vi "Get generated report  n log in sql.vi"() -> ()   [LabVIEW 2017]
uses:
  SQL/SQL/SQL_DB-Enum.ctl
  Detailed Report/Controls/Detailed_Reports_Columns.ctl
  <vilib>/Utility/error.llb/whitespace.ctl
  <vilib>/Utility/file.llb/Read Delimited Spreadsheet (string).vi
  <vilib>/addons/database/Auxilliary.llb/DB Tools DataTypes.ctl
  <vilib>/addons/database/NI_Database_API.lvlib
  SQL/Detailed Report _Colums_Informatin.ctl
  <vilib>/addons/database/Auxilliary.llb/DB Tools Parameter Dir.ctl
  <vilib>/addons/database/Auxilliary.llb/DB Tools Parameter Info.ctl
panel:
  out "error in (no error) 3":errorcluster
  out "Array":T1(array[cluster])
  in  "time stamp":timestamp
  out "Data out 2":string[][](array[string])
  out "Table/Columns":string[](array[string])
  out "size(s) 3":i32
  out "size(s) 2":i32
  out "size(s)":i32[](array[numeric])
  out "error in (no error) 2":errorcluster
  in  "error in (no error)":errorcluster
  in  "file path (dialog if empty)":path
  out "Serial Number":string
  out "Result for SQl Without Header 2":string[][](array[string])
  out "Result wiht Header 2":string[][](array[string])
  in  "User Name 2":string="mmk"
  in  "Shift 2":string="A"
  in  "Test Type 2":string="Test type"
  in  "Excepted Value 2":string="Excepted Value"
  out "Application Verision":string
  out "Variant":string
  out "Model":string
  out "all rows 2":string[][](array[string])
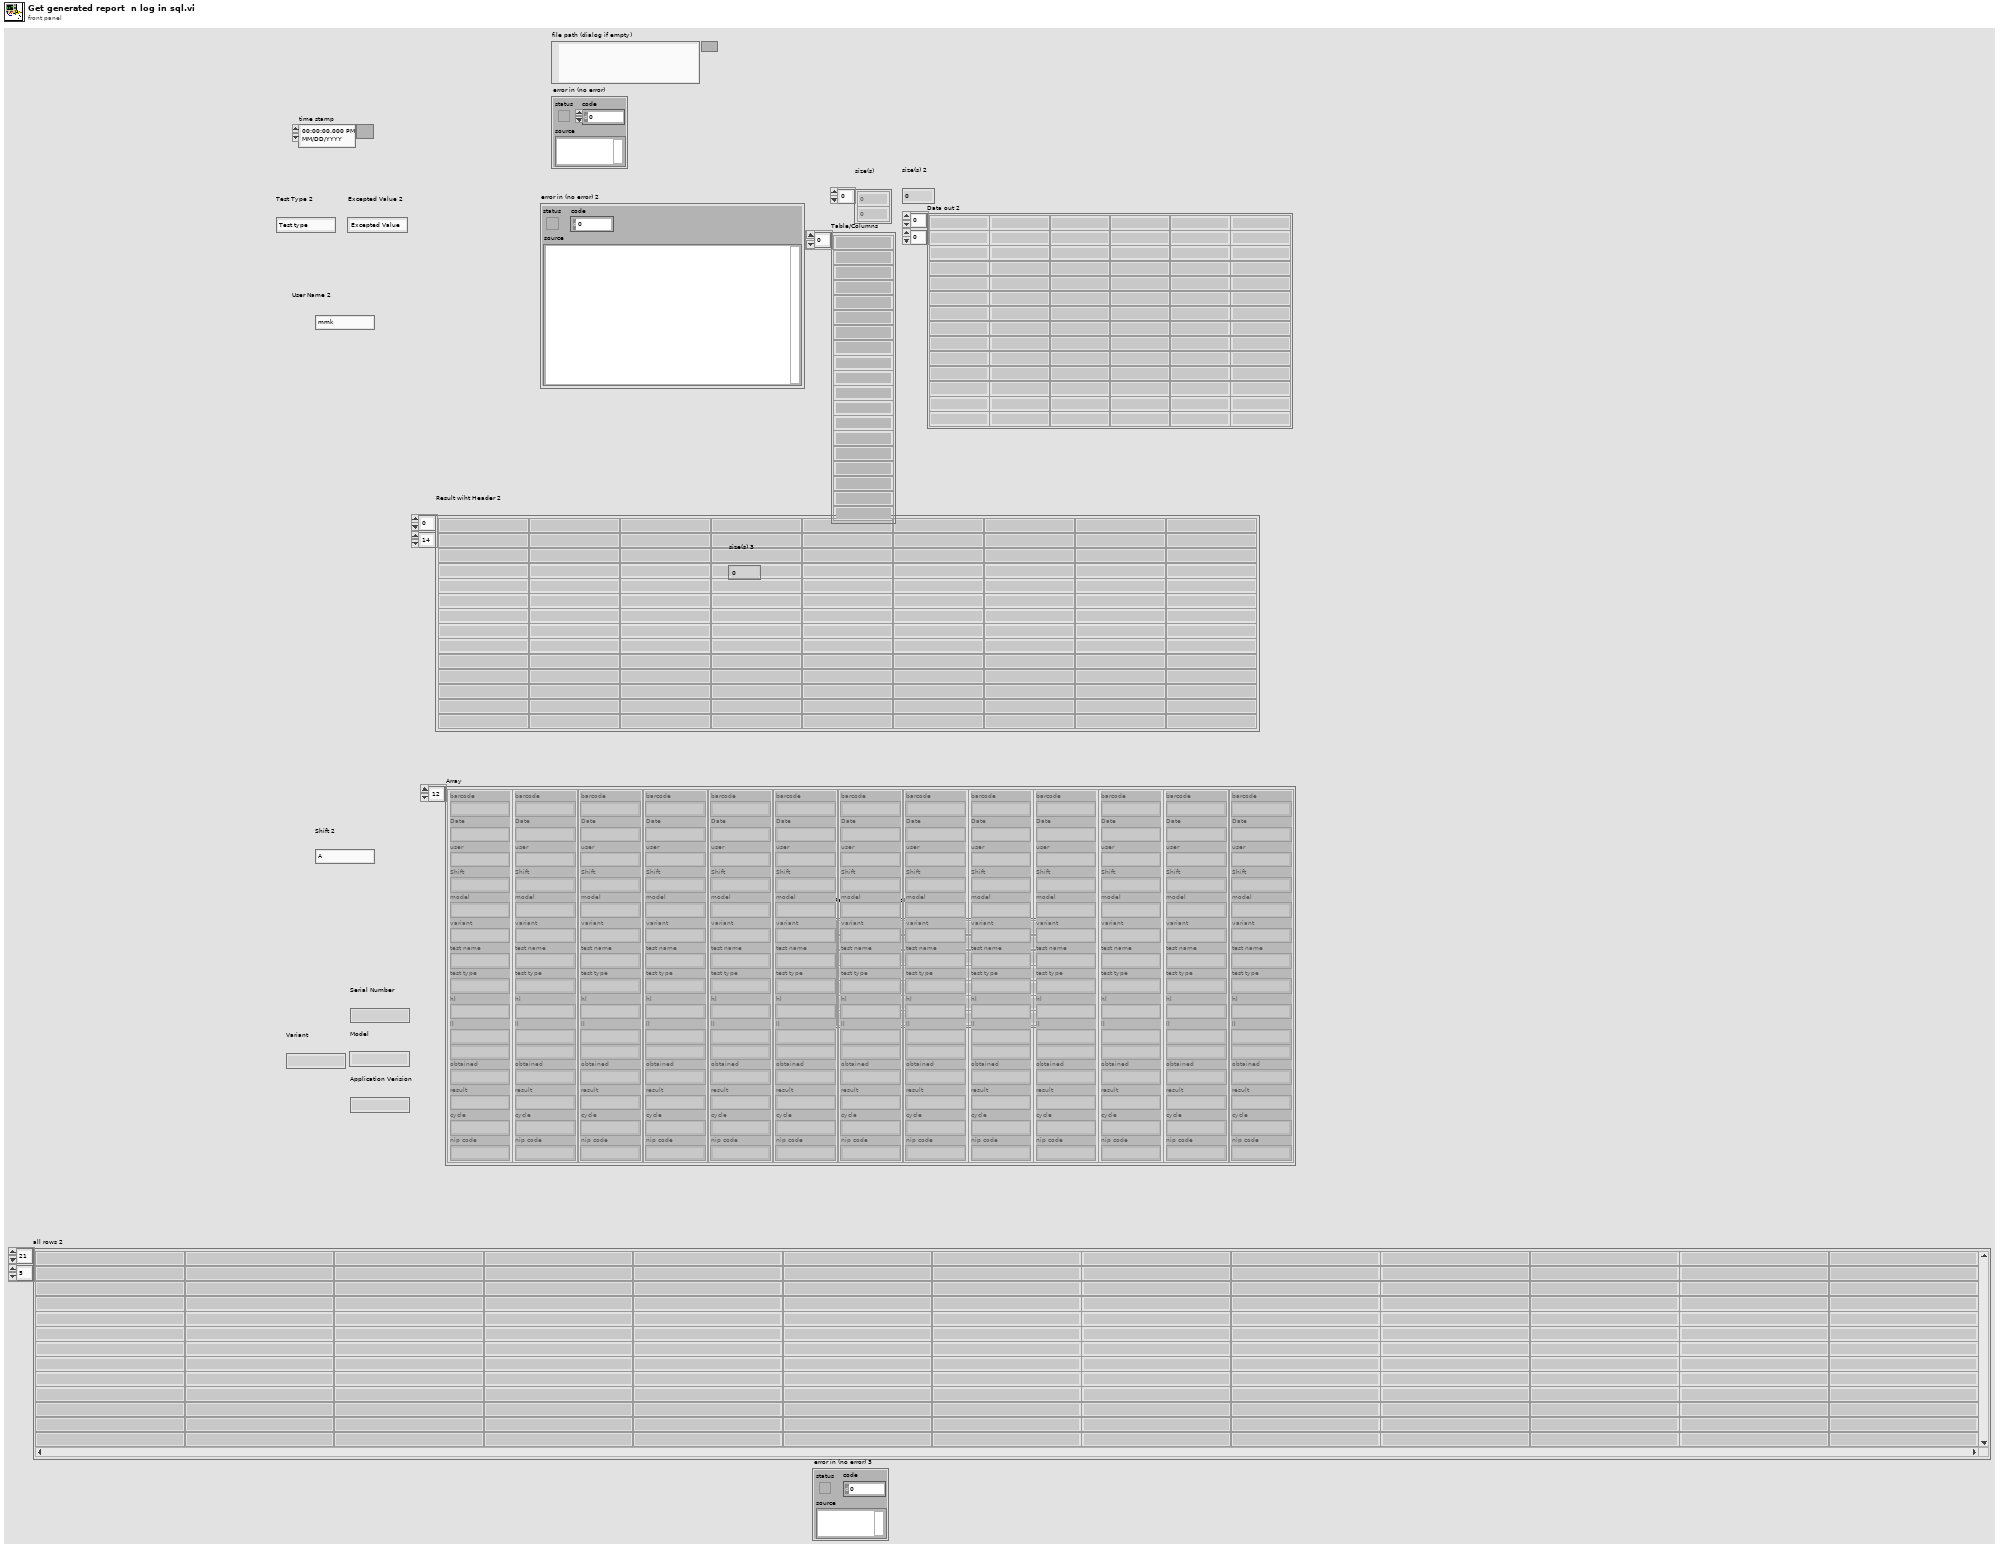
[diagram p1: front panel]
types:
  T1 = cluster{"barcode":string, "Date":string, "user":string, "Shift":string, "model":string, "variant":string, "test name":string, "test type":string, "hl":string, "ll":string, string, "obtained":string, "result":string, "cycle":string, "nip code":string}[]
  T2 = typedef "NI_Database_API.lvlib/DB Tools Parameter Info.ctl" = cluster{"parameter name":string, "type":T3, "direction":T4, "value":variant}
  T3 = typedef "NI_Database_API.lvlib/DB Tools DataTypes.ctl" = enum16{"String", "Long (I32)", "Single (SGL)", "Double (DBL)", "Date/Time", "Binary"}
  T4 = typedef "NI_Database_API.lvlib/DB Tools Parameter Dir.ctl" = enum32{"Input", "Output", "Input/Output", "Return Value"}
  T5 = typedef "SQL_DB-Enum.ctl" = enum16{"INI DATA", "Open Connections", "Query", "Update Table", "Get Full Report", "Get Serial Numbers", "Get Table Columns", "Get Table Names", "Check & Create Table", "Close Connection"}
  T6 = cluster{"barcode":string, "Date":string, "user":string, "Shift":string, "model":string, "variant":string, "test name":string, "test type":string, "hl":string, "ll":string, string, "obtained":string, "result":string, "cycle":string, "nip code":string}
  T7 = cluster{string, string, string, string, string, string, string, string, string, string, string, string, string, string, string}
  T8 = typedef "Detailed Report _Colums_Informatin.ctl" = cluster{"column name":string, "data type":T3, "size":i32, "allow null?":bool}[]
  T9 = typedef "Detailed_Reports_Columns.ctl" = string[]
  T10 = typedef "whitespace.ctl" = u16
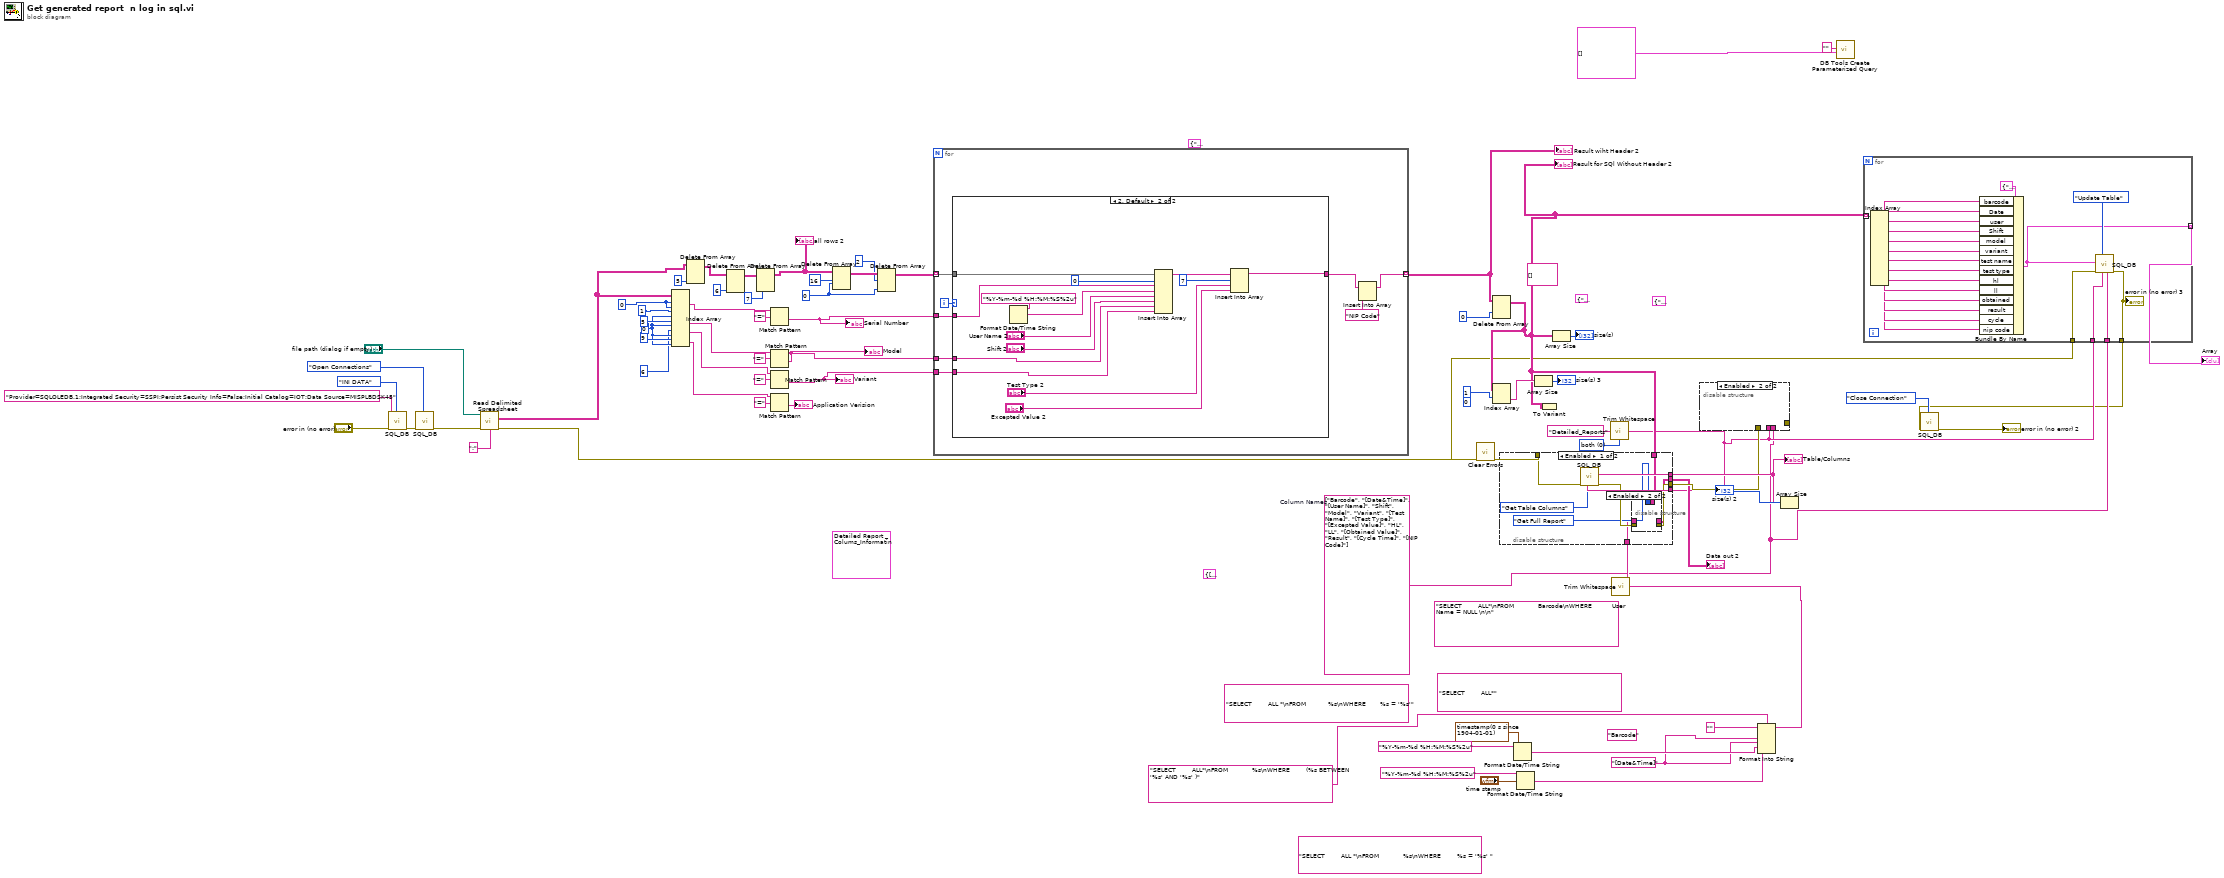
[diagram p0: block diagram]
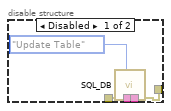
[diagram p2: hidden frame]
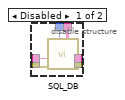
[diagram p3: hidden frame]
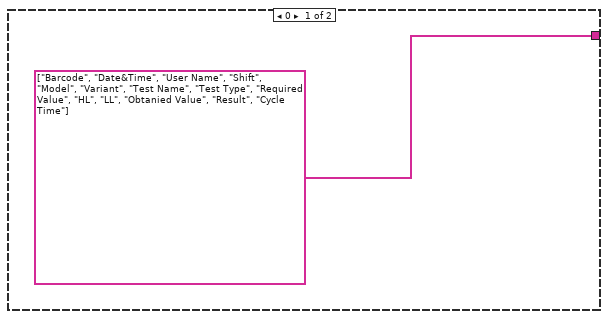
[diagram p5: hidden frame]
diagram:
  (unwired) T6 {"barcode"="barcode", "Date"="2019-12-13 20:24:09.05", "user"="1", "Shift"="shifr", "model"="model", "variant"="variant", "test name"="test name", "test type"="test type", "hl"="hl", "ll"="ll", "shifr", "obtained"="obtained", "result"="resrut", "cycle"="Cycle time", "nip code"="nip code"}
  (unwired) string[][] [] ("array w/ subset deleted")
  (unwired) T6 {"barcode"="barcode", "Date"="2019-12-13 20:24:09.05", "user"="1", "Shift"="shifr", "model"="model", "variant"="variant", "test name"="test name", "test type"="test type", "hl"="hl", "ll"="ll", "shifr", "obtained"="obtained", "result"="resrut", "cycle"="Cycle time", "nip code"="nip code"}
  (unwired) T7 {"barcode", "2019-12-13 20:24:09.05", "1", "shifr", "model", "variant", "test name", "test type", "hl", "ll", "shifr", "obtained", "resrut", "Cycle time", "nip code"}
  (unwired) "SELECT        ALL *\nFROM            %s\nWHERE        %s = '%s' "
  w10 = "[Date&Time]"
  (unwired) "Barcode"
  (unwired) "SELECT        ALL*\nFROM            Barcode\nWHERE          User Name = NULL \n\n"
  (unwired) "SELECT        ALL *\nFROM           %s\nWHERE       %s = '%s'"
  (unwired) "SELECT        ALL*"
  (unwired) T8 [{"column name"="Barcode", "data type"=enum."String", "size"=50, "allow null?"=FALSE}, {"column name"="[Date&Time]", "data type"=enum."Date/Time", "size"=50, "allow null?"=FALSE}, {"column name"="[User Name]", "data type"=enum."String", "size"=50, "allow null?"=FALSE}, {"column name"="Shift", "data type"=enum."String", "size"=50, "allow null?"=FALSE}, {"column name"="Model", "data type"=enum."String", "size"=50, "allow null?"=FALSE}, {"column name"="Variant", "data type"=enum."String", "size"=50, "allow null?"=FALSE}, {"column name"="[Test Name]", "data type"=enum."String", "size"=50, "allow null?"=FALSE}, {"column name"="[Test Type]", "data type"=enum."String", "size"=50, "allow null?"=FALSE}, {"column name"="[Excepted Value]", "data type"=enum."String", "size"=50, "allow null?"=FALSE}, {"column name"="HL", "data type"=enum."String", "size"=10, "allow null?"=FALSE}, {"column name"="LL", "data type"=enum."String", "size"=10, "allow null?"=FALSE}, {"column name"="[Obtained Value]", "data type"=enum."String", "size"=50, "allow null?"=FALSE}, {"column name"="Result", "data type"=enum."String", "size"=10, "allow null?"=FALSE}, {"column name"="[Cycle Time]", "data type"=enum."String", "size"=10, "allow null?"=FALSE}, {"column name"="[NIP Code]", "data type"=enum."String", "size"=15, "allow null?"=FALSE}] ("Array 2")
  (unwired) cluster{string[]} {["", "", "", "", "", "", "", "", "", "", "", "0", "0", "0"]}
  w6 = T9 ["Barcode", "[Date&Time]", "[User Name]", "Shift", "Model", "Variant", "[Test Name]", "[Test Type]", "[Excepted Value]", "HL", "LL", "[Obtained Value]", "Result", "[Cycle Time]", "[NIP Code]"]  # Column Names
  w28 = T10 0 items=["both", "start of string", "end of string"] ("location (both)")
  (unwired) 0 ("disabled index (col)")
  w59 = 0 ("index (row)")
  w50 = 0 ("disabled index (col)")
  w53 = 0 ("disabled index (col)")
  n1 = call "SQL_DB.vi"("CTRL"=SQL_DB-Enum."INI DATA", "error in (no error)"="error in (no error)", "Connection Info"="Provider=SQLOLEDB.1;Integrated Security=SSPI;Persist Security Info=False;Initial Catalog=IOT;Data Source=MISPLBDSK45") -> ("error in (no error) 2"=w35:errorcluster)  [unwired: 6 in, 2 out]
  n2 = call "SQL_DB.vi"("CTRL"=SQL_DB-Enum."Open Connections", "error in (no error)"=w35) -> ("error in (no error) 2"=w34:errorcluster)  [unwired: 7 in, 2 out]
  n3 = call-poly <vilib>:"Read Delimited Spreadsheet.vi"("file path (dialog if empty)"="file path (dialog if empty)", "error in (no error)"=w34, "delimiter (\\t)"=":" ("delimiter (\\t)")) -> ("all rows"=w42:string[][], "error out"=w33:errorcluster)  [unwired: 7 in, 4 out]
  n4 = Index Array(array=w42, index (row) #1=w59, index (col) #1=w59, index (row) #2=1 ("index (row)"), index (col) #2=w53, index (row) #3=5 ("index (row)"), index (col) #3=w53, index (row) #4=6 ("index (row)"), index (col) #4=w53, index (row) #5=9 ("index (row)"), index (col) #5=w53) -> (element #1=w57:string, element #3=w70:string, element #4=w67:string, element #5=w63:string)  [unwired: 1 out]
  n5 = Delete From Array(array=w42, index (col)=5 ("disabled index (col)")) -> (array with subset deleted=w41:string[][])  [unwired: 2 in, 1 out]
  n6 = Delete From Array(array=w41, index (col)=6 ("disabled index (col)")) -> (array with subset deleted=w47:string[][])  [unwired: 2 in, 1 out]
  n7 = Delete From Array(array=w47, index (col)=7 ("disabled index (col)")) -> (array with subset deleted=w46:string[][])  [unwired: 2 in, 1 out]
  "all rows 2" <- w46
  n8 = Match Pattern(string=w70, regular expression="=") -> (after substring=w55:string)  [unwired: 1 in, 3 out]
  "Model" <- w55
  n9 = Match Pattern(string=w67, regular expression="=") -> (after substring=w54:string)  [unwired: 1 in, 3 out]
  "Variant" <- w54
  n10 = Match Pattern(string=w57, regular expression="=") -> (after substring=w56:string)  [unwired: 1 in, 3 out]
  "Serial Number" <- w56
  n11 = Match Pattern(string=w63, regular expression="=") -> (after substring=→"Application Verision":string)  [unwired: 1 in, 3 out]
  n12 = Delete From Array(array=w46, length=16, index (row)=w50) -> (array with subset deleted=w51:string[][])  [unwired: 1 in, 1 out]
  n13 = Delete From Array(array=w51, length=2, index (col)=w50) -> (array with subset deleted=w48:string[][])  [unwired: 1 in, 1 out]
  n14 = for {
    tunnel: w48 -> [w80] mode=indexing
    tunnel: [w73] -> w61 mode=indexing
    tunnel: w56 -> [w78]
    tunnel: w55 -> [w77]
    tunnel: w54 -> [w76]
    i -> [w79]
    n15 = case shown="2, Default" w79 {
      tunnel: w80 -> [_ w95]
      tunnel: [string[] ["Barcode", "Date&Time", "User Name", "Shift", "Model", "Variant", "Test Name", "Test Type", "Required Value", "HL", "LL", "Obtanied Value", "Result", "Cycle Time"] w87] -> w75
      tunnel: w78 -> [_ w84]
      tunnel: w77 -> [_ w83]
      tunnel: w76 -> [_ w82]
      frame 0 {
      }
      frame 2, Default {
        n16 = Format Date/Time String(time format string (%c)="%Y-%m-%d %H:%M:%S%2u") -> (date/time string=w85:string)  [unwired: 2 in]
        n17 = Insert Into Array(array=w95, index=0, new element #1=w84, new element #2=w85, new element #3="User Name 2", new element #4="Shift 2", new element #5=w83, new element #6=w82) -> (w91:string[])
        n18 = Insert Into Array(array=w91, index=7, new element #1="Test Type 2", new element #2="Excepted Value 2") -> (w87:string[])
      }
    }
    n19 = Insert Into Array(array=w75, new element="NIP Code" ("new element/subarray")) -> (w73:string[])  [unwired: 1 in]
  }
  "Result wiht Header 2" <- w61
  n20 = call <vilib>:"Clear Errors.vi"("error in (no error)"=w33) -> ("error out"=w3:errorcluster)  [unwired: 5 in, 1 out]
  n21 = Delete From Array(array=w61, index (row)=0 ("disabled index (col)")) -> (array with subset deleted=w8:string[][])  [unwired: 2 in, 1 out]
  "Result for SQl Without Header 2" <- w8
  n22 = Index Array(array=w8, index (row)=1 ("length")) -> (element=w23:string[])  [unwired: 1 in]
  n23 = Format Date/Time String(time format string (%c)="%Y-%m-%d %H:%M:%S%2u", seconds (now)=timestamp(0 s since 1904-01-01) ("time stamp")) -> (date/time string=w13:string)  [unwired: 1 in]
  n24 = Format Date/Time String(time format string (%c)="%Y-%m-%d %H:%M:%S%2u", seconds (now)="time stamp") -> (date/time string=w12:string)  [unwired: 1 in]
  n25 = Array Size(array=w23) -> (size(s)=→"size(s) 3":i32)
  n26 = To Variant(anything=w8) -> ()  [unwired: 1 out]
  n27 = Array Size(array=w8) -> (size(s)=→"size(s)":i32[])
  n28 = call <vilib>:"Trim Whitespace.vi"("string"="Detailed_Reports" ("Table Name"), "location (both)"=w28) -> ("trimmed string"=w7:string)
  n29 = Format Into String(format string="SELECT        ALL*\nFROM            %s\nWHERE        (%s BETWEEN  '%s' AND '%s' )", initial string="", w10, w10, w13, w12) -> (resulting string=w15:string)  [unwired: 1 in, 1 out]
  n30 = call <vilib>:"Trim Whitespace.vi"("string"=w15) -> ("trimmed string"=w20:string)  [unwired: 1 in]
  n31 = disable-structure shown="Enabled" {
    disable-tunnel: w3 -> [w105 w112]
    disable-tunnel: w7 -> [w104 _]
    disable-tunnel: [w103 _] -> w24
    disable-tunnel: [w100 w112] -> w22
    disable-tunnel: [w98 _] -> w21
    disable-tunnel: w20 -> [w97 _]
    disable-tunnel: w8 -> [w96 _]
    frame Enabled {
      n32 = call "SQL_DB.vi"("Table Name"=w104, "CTRL"=SQL_DB-Enum."Get Table Columns", "error in (no error)"=w105) -> ("error in (no error) 2"=w101:errorcluster, "Table/Columns"=w103:string[])  [unwired: 6 in, 1 out]
      n33 = disable-structure shown="Enabled" {
        disable-tunnel: w101 -> [w111 _]
        disable-tunnel: [w110 _] -> w100
        disable-tunnel: SQL_DB-Enum."Get Full Report" ("CTRL") -> [w109 _]
        disable-tunnel: [w108 _] -> w98
        disable-tunnel: w97 -> [w107 _]
        disable-tunnel: w96 -> [w106 _]
        frame Disabled {
          n34 = call "SQL_DB.vi"("datatype"=w106, "CTRL"=w109, "error in (no error)"=w111, "SQL query"=w107) -> ("error in (no error) 2"=w110:errorcluster, "Data out 2"=w108:string[][])  [unwired: 5 in, 1 out]
        }
        frame Enabled {
        }
      }
    }
    frame Disabled {
    }
  }
  "Table/Columns" <- w24
  "Data out 2" <- w21
  n35 = disable-structure shown="Enabled" {
    disable-tunnel: [w117 _] -> _
    disable-tunnel: w22 -> [w116 _]
    disable-tunnel: w7 -> [w114 _]
    disable-tunnel: w6 -> [w113 _]
    frame Disabled {
      n36 = call "SQL_DB.vi"("Column Names"=w113, "Table Name"=w114, "CTRL"=SQL_DB-Enum."Update Table", "error in (no error)"=w116) -> ("error in (no error) 2"=w117:errorcluster)  [unwired: 5 in, 2 out]
    }
    frame Enabled {
    }
  }
  n37 = Array Size(array=w24) -> (size(s)=→"size(s) 2":i32)
  n38 = call <vilib>:"DB Tools Create Parameterized Query.vi"("parameters"=T2[] [], "SQL query"="") -> ()  [unwired: 5 in, 3 out]
  n39 = for {
    tunnel: w8 -> [w139] mode=indexing
    tunnel: [w120] -> w9 mode=indexing
    tunnel: w7 -> [w122]
    tunnel: w6 -> [w121]
    tunnel: [w119] -> w4
    tunnel: w3 -> [w118]
    n40 = Index Array(array=w139) -> (element #1=w137:string, element #2=w136:string, element #3=w135:string, element #4=w134:string, element #5=w133:string, element #6=w132:string, element #7=w131:string, element #8=w130:string, element #9=w129:string, element #10=w128:string, element #11=w127:string, element #12=w126:string, element #13=w125:string, element #14=w124:string)  [unwired: 14 in]
    n41 = Bundle By Name(cluster=T6 {"barcode"="barcode", "Date"="2019-12-13 20:24:09.05", "user"="1", "Shift"="shifr", "model"="model", "variant"="variant", "test name"="test name", "test type"="test type", "hl"="hl", "ll"="ll", "shifr", "obtained"="obtained", "result"="resrut", "cycle"="Cycle time", "nip code"="nip code"}, "barcode"=w137, "Date"=w136, "user"=w135, "Shift"=w134, "model"=w133, "variant"=w132, "test name"=w131, "test type"=w130, "hl"=w129, "ll"=w128, "obtained"=w127, "result"=w126, "cycle"=w125, "nip code"=w124) -> (w120:T6)
    n42 = call "SQL_DB.vi"("Column Names"=w121, "Table Name"=w122, "CTRL"=SQL_DB-Enum."Update Table", "error in (no error)"=w118, "data to Update"=w120) -> ("error in (no error) 2"=w119:errorcluster)  [unwired: 4 in, 2 out]
    "error in (no error) 3" <- w119
  }
  "Array" <- w9
  n43 = call "SQL_DB.vi"("CTRL"=SQL_DB-Enum."Close Connection", "error in (no error)"=w4) -> ("error in (no error) 2"=→"error in (no error) 2":errorcluster)  [unwired: 7 in, 2 out]
